vi "elimina collaudo.vi"(6 "table":string, 7 "anno":string, 8 "banco":string, 9 "tipo prova":string, 10 "progressivo":string, 11 "Refnum in":T1) -> (3 "Refnum out":T1)   [LabVIEW 2019]
uses:
  <vilib>/addons/database/Connection.llb/Conn ObjectReference.ctl
  <vilib>/addons/database/NI_Database_API.lvlib
panel:
  out "concatenated string":string
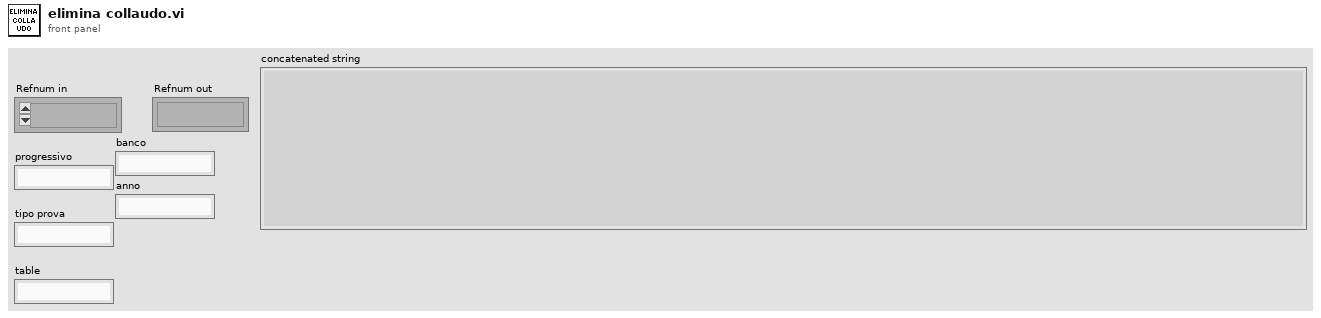
[diagram p1: front panel]
types:
  T1 = typedef "NI_Database_API.lvlib/Conn ObjectReference.ctl" = refnum<k1>
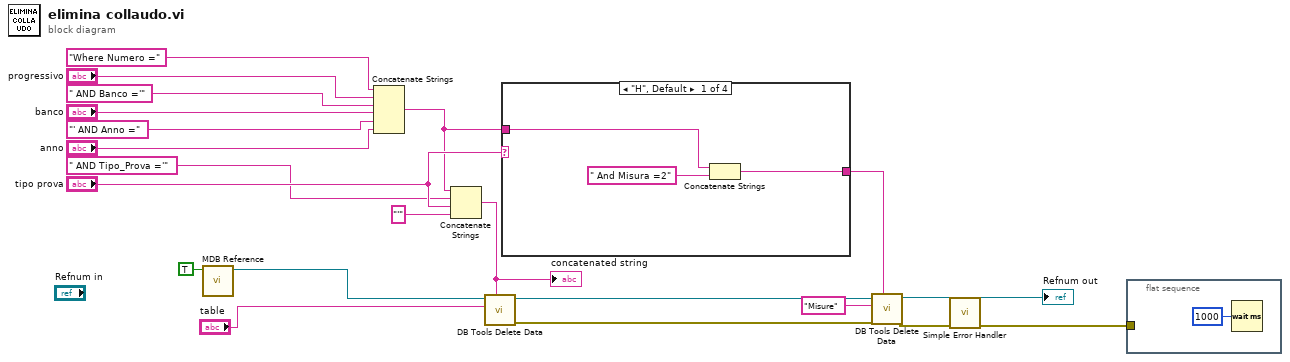
[diagram p0: block diagram]
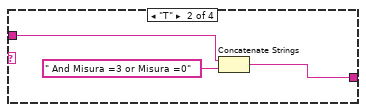
[diagram p2: hidden frame]
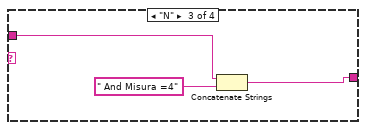
[diagram p3: hidden frame]
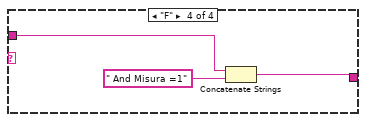
[diagram p4: hidden frame]
diagram:
  n1 = call "MDB Reference.vi"("Collaudi T/motori F"=TRUE ("NM?")) -> ("Refnum out"=w2:T1)  [unwired: 8 in, 2 out]
  n2 = Concatenate Strings("Where Numero =" ("condition"), "progressivo", " AND Banco ='" ("string"), "banco", "' AND Anno =" ("string"), "anno") -> (w8:string)
  n3 = Concatenate Strings(w8, " AND Tipo_Prova ='" ("string"), "tipo prova", "'" ("string")) -> (w15:string)
  "concatenated string" <- w15
  n4 = call <vilib>:"DB Tools Delete Data.vi"("condition"=w15, "table"="table", "connection reference"=w2) -> ("error out"=w11:errorcluster, "connection reference out"=w20:T1)  [unwired: 7 in]
  n5 = case shown="\"H\", Default" "tipo prova" {
    tunnel: w8 -> [w24 w26 w29 w32]
    tunnel: [w23 w25 w28 w31] -> w12
    frame "H", Default {
      n6 = Concatenate Strings(w24, " And Misura =2" ("string")) -> (w23:string)
    }
    frame "T" {
      n7 = Concatenate Strings(w26, " And Misura =3 or Misura =0" ("string")) -> (w25:string)
    }
    frame "N" {
      n8 = Concatenate Strings(w29, " And Misura =4" ("string")) -> (w28:string)
    }
    frame "F" {
      n9 = Concatenate Strings(w32, " And Misura =1" ("string")) -> (w31:string)
    }
  }
  n10 = call <vilib>:"DB Tools Delete Data.vi"("condition"=w12, "error in (no error)"=w11, "table"="Misure", "connection reference"=w20) -> ("error out"=w10:errorcluster, "connection reference out"=→"Refnum out":T1)  [unwired: 6 in]
  n11 = call <vilib>:"Simple Error Handler.vi"("error in (no error)"=w10) -> ("error out"=w1:errorcluster)  [unwired: 4 in, 4 out]
  n12 = flat-sequence {
    tunnel: w1 -> [_]
    frame #0 {
      n13 = Wait (ms)(milliseconds to wait=u32 1000) -> ()  [unwired: 1 out]
    }
  }
